vi "Write Scope.vi"(10 "Scope":T1, 11 "Attribute in":refnum<class "Attribute.lvclass">) -> (3 "Attribute out":refnum<class "Attribute.lvclass">)   [LabVIEW 2013, in "Attribute.lvclass"]
uses:
  Attribute.lvclass
  Definitions/def.SMO/Scope -- Enum.ctl
  Attribute.lvclass/Attribute.ctl
  Definitions/def.SMO/def.SMO.lvclass
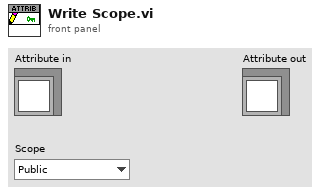
[diagram p1: front panel]
types:
  T1 = typedef "def.SMO.lvclass/Scope -- Enum.ctl" = enum16{"Public", "Protected", "Private"}
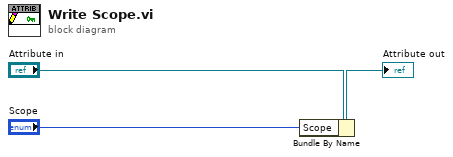
[diagram p0: block diagram]
diagram:
  n1 = Bundle By Name(cluster="Attribute in", "Scope"="Scope") -> (→"Attribute out":refnum<class "Attribute.lvclass">)
